vi "Target Frame Period.vi"() -> (3 "Target Frame Period [ms]":u32)   [LabVIEW 2015]
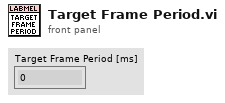
[diagram p1: front panel]
types:
  T1 = typedef "Constants.ctl" = cluster{"Colours":cluster{"OK":u32, "Warning":u32, "Error":u32, "Green On":u32, "Green Off":u32, "Red On":u32, "Red Off":u32}, "System":cluster{"Target Frames Second":dbl, "Field Size":T2}}
  T2 = typedef "Math.lvlib/Point (SGL).ctl" = cluster{"x":sgl, "y":sgl}
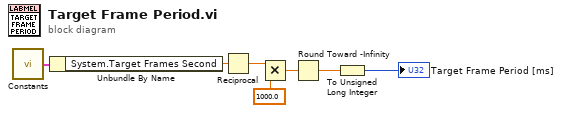
[diagram p0: block diagram]
diagram:
  n1 = call "Constants.vi"() -> ("Constants"=w4:T1)
  n2 = Unbundle By Name(w4) -> ("System.Target Frames Second"=w5:dbl)
  n3 = Reciprocal(x=w5) -> (1/x=w6:dbl)
  n4 = Multiply(x=w6, y=1000.0) -> (x*y=w3:dbl)
  n5 = Round Toward -Infinity(1:w3) -> (0:w2:dbl)
  n6 = To Unsigned Long Integer(number=w2) -> (unsigned 32bit integer=→"Target Frame Period [ms]":u32)
